vi "Release Session.vi"(8 "error in (no error)":errorcluster, 11 "session":T1) -> (0 "error out":errorcluster)   [LabVIEW 2017, in "libssh2.lvlib"]
uses:
  libssh2.lvlib
  Session Refnum.ctl
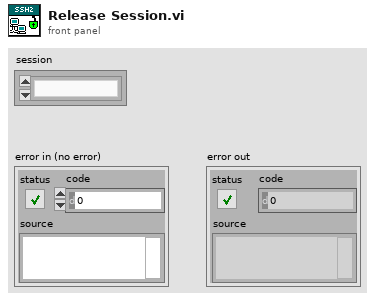
[diagram p1: front panel]
types:
  T1 = typedef "libssh2.lvlib/Session Refnum.ctl" = refnum<k1>
  T2 = typedef "Semaphore RefNum" = refnum<k1>
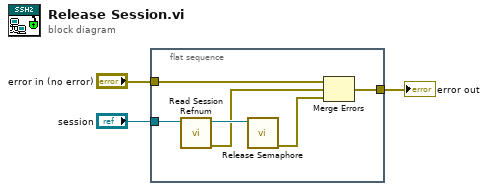
[diagram p0: block diagram]
diagram:
  n1 = flat-sequence {
    tunnel: [w6] -> w3
    tunnel: "error in (no error)" -> [w5]
    tunnel: "session" -> [w4]
    frame #0 {
      n2 = call "Read Session Refnum.vi"("session"=w4) -> ("error out"=w8:errorcluster, "semaphore"=w9:T2)  [unwired: 5 in, 4 out]
      n3 = call <vilib>:"Release Semaphore.vi"("semaphore"=w9) -> ("error out"=w7:errorcluster)  [unwired: 5 in, 1 out]
      n4 = Merge Errors(w5, w8, w7) -> (w6:errorcluster)
    }
  }
  "error out" <- w3
